vi "_044.vi"() -> ()   [LabVIEW 2024]
panel:
  out "Boolean 12":bool
  in  "Boolean 11":bool
  out "Boolean 10":bool
  in  "Boolean 9":bool
  out "Boolean 8":bool
  in  "Boolean 7":bool
  out "Boolean 6":bool
  in  "Boolean 5":bool
  out "Boolean 4":bool
  in  "Boolean 3":bool
  out "Boolean 2":bool
  in  "Boolean":bool
  # "Mechanical Actions :"
  # "Switch when pressed :"
  # "Latch when pressed :"
  # "Switch when released :"
  # "Latch when released :"
  # "Switch until released :"
  # "Latch until released :"
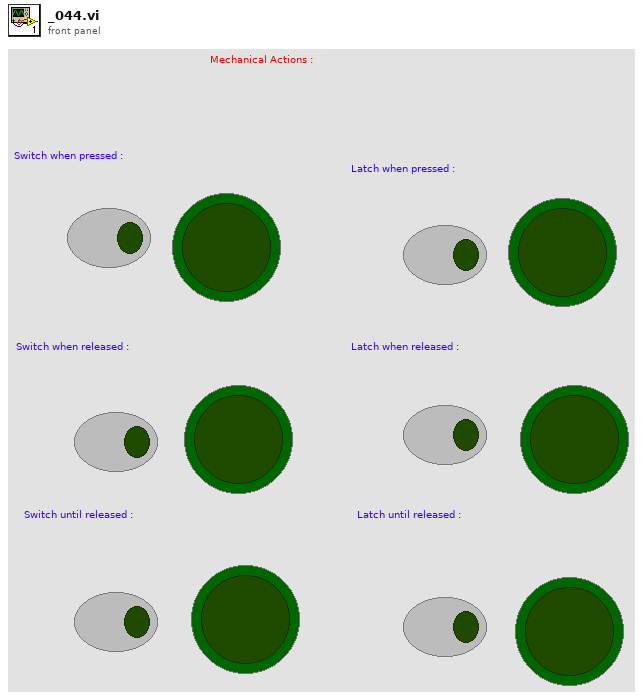
[diagram p1: front panel]
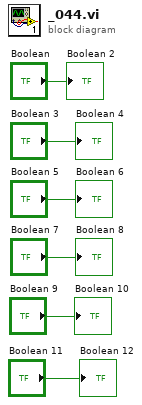
[diagram p0: block diagram]
diagram:
  "Boolean 2" <- "Boolean"
  "Boolean 4" <- "Boolean 3"
  "Boolean 6" <- "Boolean 5"
  "Boolean 8" <- "Boolean 7"
  "Boolean 10" <- "Boolean 9"
  "Boolean 12" <- "Boolean 11"
